vi "Read String.vi"(8 "error in (no error)":errorcluster, 11 "ListboxEditCellMsg in":refnum<class "ListboxEditCellMsg.lvclass">) -> (0 "error out":errorcluster, 2 "String":string, 3 "ListboxEditCellMsg out":refnum<class "ListboxEditCellMsg.lvclass">)   [LabVIEW 2015, in "ActorEvents.lvlib" / "ListboxEditCellMsg.lvclass"]
uses:
  ListboxEditCellMsg.lvclass
  ListboxEditCellMsg.lvclass/ListboxEditCellMsg.ctl
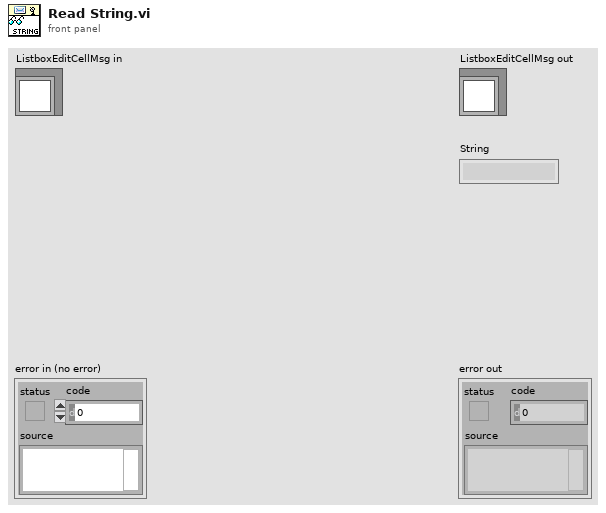
[diagram p1: front panel]
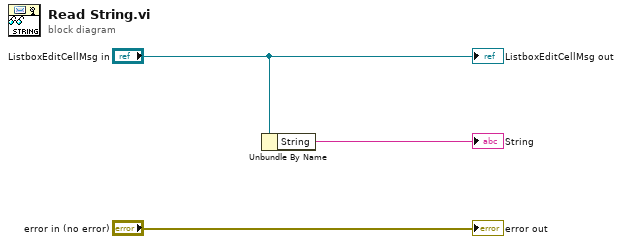
[diagram p0: block diagram]
diagram:
  n1 = Unbundle By Name("ListboxEditCellMsg in") -> ("String"=→"String":string)
  "error out" <- "error in (no error)"
  "ListboxEditCellMsg out" <- "ListboxEditCellMsg in"
